vi "Watch Dog Read.vi"(9 "Time Out":dbl, 11 "Read Array":string[](array[string])) -> (1 "Time Out":bool)   [LabVIEW 2015]
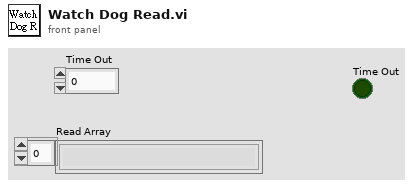
[diagram p1: front panel]
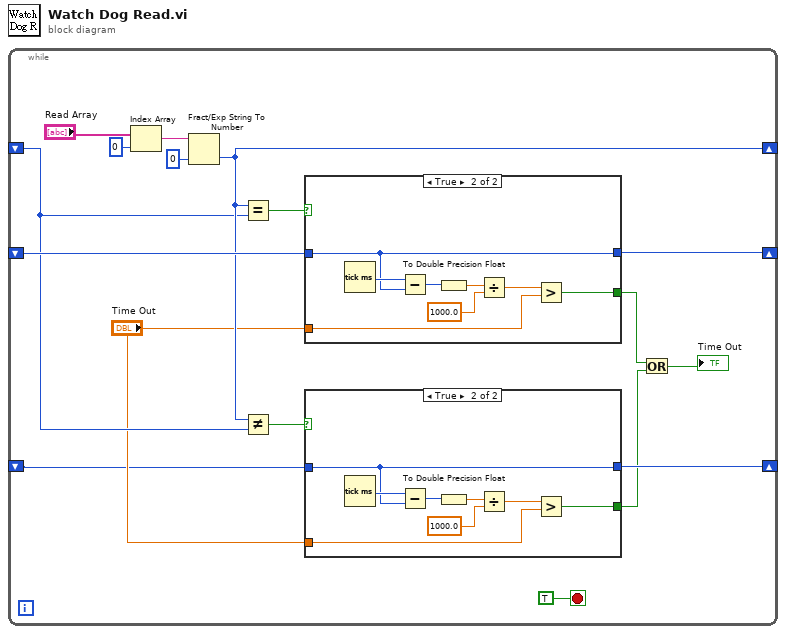
[diagram p0: block diagram]
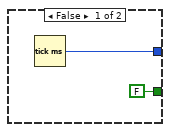
[diagram p2: hidden frame]
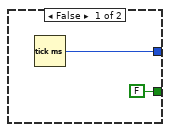
[diagram p3: hidden frame]
diagram:
  n1 = while {
    shift-right: [w8] -> _
    shift-left: _ -> [w7]
    shift-right: [w14] -> _
    shift-left: _ -> [w13]
    shift-right: [w5] -> _
    shift-left: _ -> [w4]
    stop <- TRUE stop-if-true
    n2 = Index Array(array="Read Array", index=0) -> (element=w11:string)
    n3 = Fract/Exp String To Number(string=w11, default (0 dbl)=i16 0 ("precision (6)")) -> (number=w8:i16)  [unwired: 2 in, 1 out]
    n4 = Equal?(x=w8, y=w7) -> (x = y?=w15:bool)
    n5 = Not Equal?(x=w8, y=w7) -> (x != y?=w9:bool)
    n6 = case shown="True" w15 {
      tunnel: [w29 w33] -> w14
      tunnel: w13 -> [_ w33]
      tunnel: "Time Out" -> [_ w31]
      tunnel: [FALSE w30] -> w3
      frame False {
        n7 = Tick Count (ms)() -> (millisecond timer value=w29:u32)
      }
      frame True {
        n8 = Tick Count (ms)() -> (millisecond timer value=w35:u32)
        n9 = Subtract(x=w35, y=w33) -> (x-y=w37:u32)
        n10 = To Double Precision Float(number=w37) -> (double precision float=w34:dbl)
        n11 = Divide(x=w34, y=1000.0) -> (x/y=w32:dbl)
        n12 = Greater?(x=w32, y=w31) -> (0:w30:bool)
      }
    }
    n13 = case shown="True" w9 {
      tunnel: [w19 w23] -> w5
      tunnel: w4 -> [_ w23]
      tunnel: "Time Out" -> [_ w21]
      tunnel: [FALSE w20] -> w2
      frame False {
        n14 = Tick Count (ms)() -> (millisecond timer value=w19:u32)
      }
      frame True {
        n15 = Tick Count (ms)() -> (millisecond timer value=w25:u32)
        n16 = Subtract(x=w25, y=w23) -> (x-y=w27:u32)
        n17 = To Double Precision Float(number=w27) -> (double precision float=w24:dbl)
        n18 = Divide(x=w24, y=1000.0) -> (x/y=w22:dbl)
        n19 = Greater?(x=w22, y=w21) -> (0:w20:bool)
      }
    }
    n20 = Or(x=w3, y=w2) -> (x .or. y?=→"Time Out":bool)
  }
